vi "Select Reference 2.vi"(1 "3D Coil":dbl[][](graph)) -> (0 "Element Data":i32)   [LabVIEW 2016]
panel:
  in  "Case Constant\n(See Context Help)":bool=TRUE
  in  "HEAD":bool
  in  "LE":bool
  in  "RE":bool
  # "Copyright Americo A. Migliaccio (c) 2002 All Rights Reserved by Author"
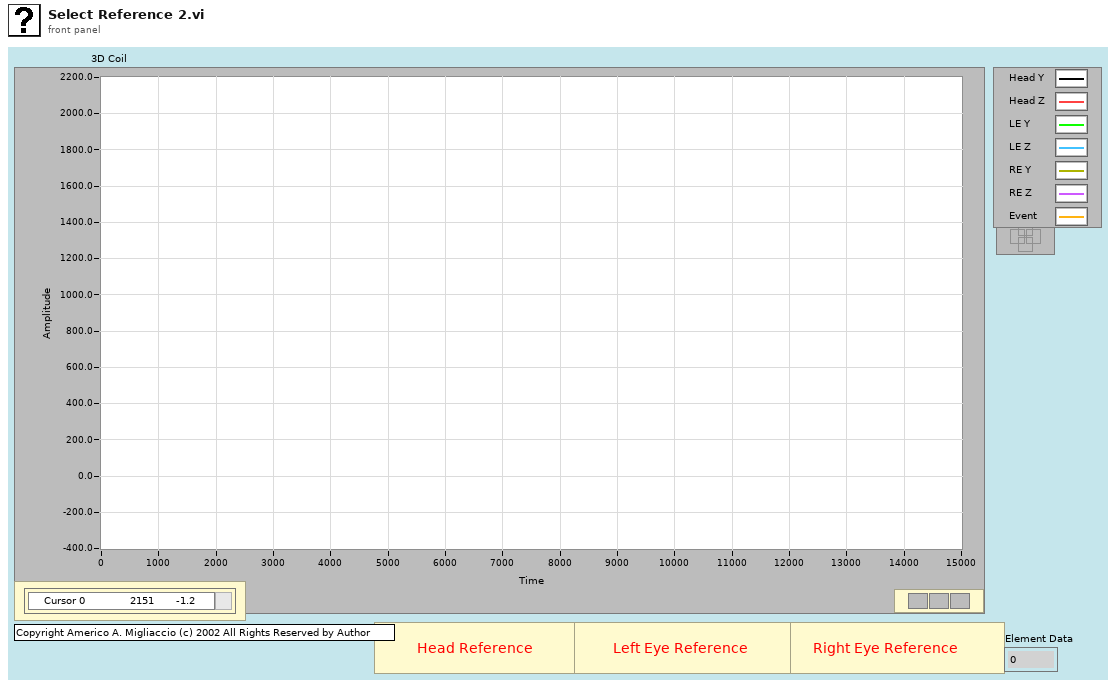
[diagram p1: front panel]
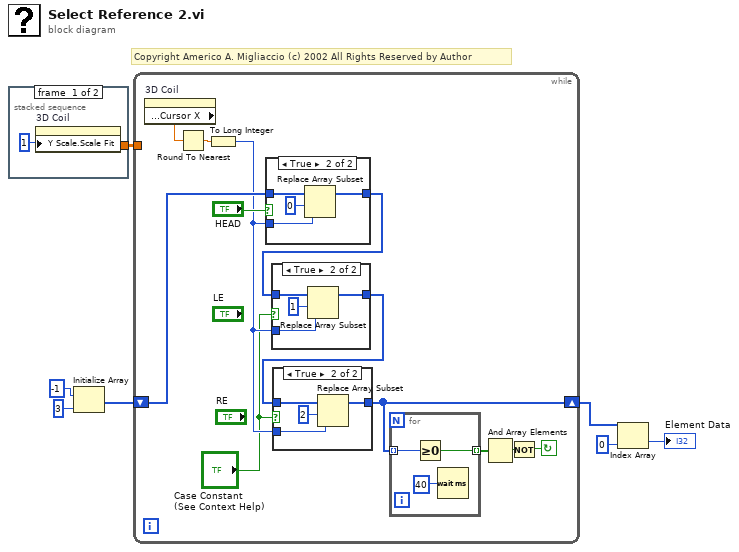
[diagram p0: block diagram]
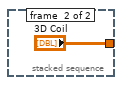
[diagram p5: hidden frame]
diagram:
  # "Copyright Americo A. Migliaccio (c) 2002 All Rights Reserved by Author"
  n1 = stacked-sequence {
    tunnel: [_ "3D Coil"] -> w7
    frame #0 {
      n2 = property on="3D Coil" class="WFGraph (strict)"("Y Scale.Scale Fit"=u8 1) -> ()  [unwired: 2 in, 2 out]
    }
    frame #1 {
    }
  }
  n3 = Initialize Array(-1 ("Element Data"), 3 ("Dimension Size")) -> (w6:i32[])
  n4 = while {
    shift-left: w6 -> [w19]
    shift-right: [w14] -> w3
    tunnel: w7 -> [_]
    stop <- w11 continue-if-true
    n5 = property on="3D Coil" class="WFGraph (strict)"() -> ("Cursor.Cursor Position:Cursor X"=w21:dbl)  [unwired: 2 in, 2 out]
    n6 = Round To Nearest(number=w21) -> (nearest integer value=w16:dbl)
    n7 = To Long Integer(number=w16) -> (32bit integer=w15:i32)
    n8 = case shown="True" "HEAD" {
      tunnel: w19 -> [w35 w38]
      tunnel: [w35 w37] -> w18
      tunnel: w15 -> [_ w36]
      frame False {
      }
      frame True {
        n9 = Replace Array Subset(array=w38, new element=w36, index=0 ("Index")) -> (w37:i32[])
      }
    }
    n10 = case shown="True" "Case Constant\n(See Context Help)" {
      tunnel: w18 -> [w30 w33]
      tunnel: [w30 w32] -> w17
      tunnel: w15 -> [_ w31]
      frame False {
      }
      frame True {
        n11 = Replace Array Subset(array=w33, new element=w31, index=1 ("Index")) -> (w32:i32[])
      }
    }
    n12 = case shown="True" "Case Constant\n(See Context Help)" {
      tunnel: w17 -> [w25 w28]
      tunnel: [w25 w27] -> w14
      tunnel: w15 -> [_ w26]
      frame False {
      }
      frame True {
        n13 = Replace Array Subset(array=w28, new element=w26, index=2 ("Index")) -> (w27:i32[])
      }
    }
    n14 = for {
      tunnel: w14 -> [w24] mode=indexing
      tunnel: [w23] -> w13 mode=indexing
      n15 = Greater Or Equal To 0?(x=w24) -> (x >= 0?=w23:bool)
      n16 = Wait (ms)(milliseconds to wait=u32 40) -> ()  [unwired: 1 out]
    }
    n17 = And Array Elements(Boolean array=w13) -> (logical AND=w12:bool)
    n18 = Not(x=w12) -> (.not. x?=w11:bool)
  }
  n19 = Index Array(array=w3, index=0) -> (element=→"Element Data":i32)
